vi "swerveData.vi"() -> ()   [LabVIEW 2019]
panel:
  out "realDistance":dbl
  out "latches[]":bool[](array[boolean])
  out "exitVI":bool
  out "finalDriveEncoders":dbl[](array[numeric])
  out "magnitudes[]":dbl[](array[numeric])
  out "steeringSings[]":dbl[](array[numeric])
  out "magnitudeMax":dbl
  out "limitSwitchs":bool[](array[boolean])
  out "RdefaultSteeringTheta":dbl[](array[numeric])
  out "LdefaultSteeringTheta":dbl[](array[numeric])
  out "final x":dbl[](array[numeric])
  out "final y":dbl[](array[numeric])
  out "finalSteeringEncoders":dbl[](array[numeric])
  out "finalGyro":dbl
  # "write: swerveTasks\nread: swerveTele"
  # "write: swerveTele\nread: swerveTele"
  # "write: swerveTele\nread: swerveTele"
  # "write: swerveTasks\nread: swerveTele"
  # "write: swerveBegin\nread: swerveTele"
  # "write: swerveBegin\nread: swerveTele"
  # "write: swerveBegin\nread: swerveTele"
  # "write: swerveBegin\nread: swerveTele"
  # "write: swerveTele\nread: swerveTasks"
  # "write: swerveTasks\nread: swerveTele"
  # "write: swerveBegin\nread: swerveTele"
  # "write: swerveTasks\nread: swerveTele"
  # "write: swerveBegin\nread: swerveTele"
  # "write: swerveTasks\nread: swerveTele"
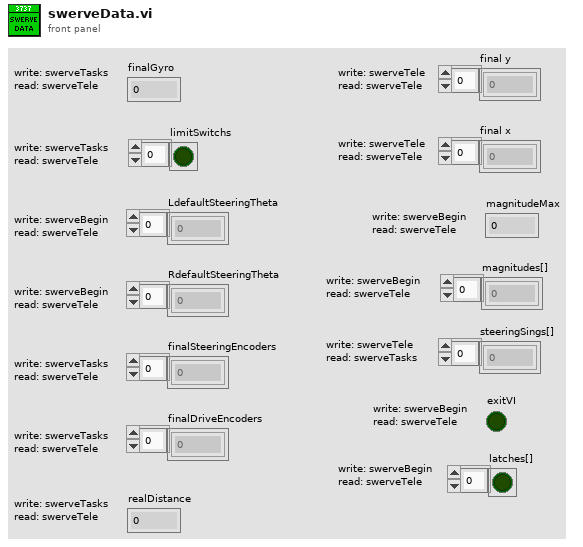
[diagram p1: front panel]
diagram:
